vi "Z Aux Set Trace File.vi"(8 "error in (no error)":errorcluster caption="错误输入（无错误）", 10 "pFilePathName":string, 11 "bifTofile":i32) -> (0 "error out":errorcluster caption="错误输出", 3 "function return":i32)   [LabVIEW 2015, in "zauxdll.lvlib"]
doc: "int32 __stdcall ZAux_SetTraceFile(int bifTofile, const char *pFilePathName);"
uses:
  zauxdll.lvlib
  Radar - 2015 32bit_autoqueue_angle_0319/zauxdll-2014/zauxdll.dll
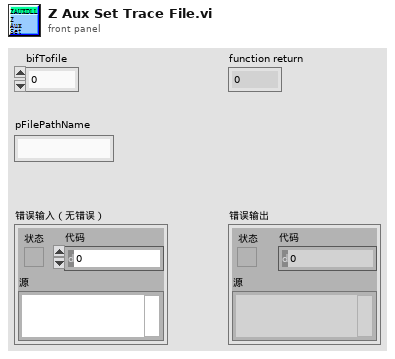
[diagram p1: front panel]
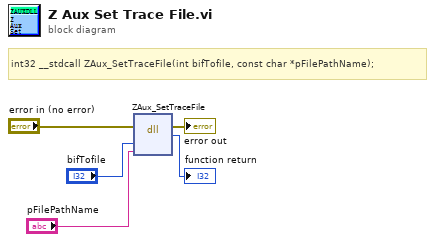
[diagram p0: block diagram]
diagram:
  # "int32 __stdcall ZAux_SetTraceFile(int bifTofile, const char *pFilePathName);"
  n1 = dll-call lib="D:/vicomm case/cub/0717/Radar - 2015 32bit_autoqueue_angle_0319/zauxdll-2014/zauxdll.*" fn="ZAux_SetTraceFile"(error in="error in (no error)", "bifTofile"="bifTofile", "pFilePathName"="pFilePathName") -> (error out=→"error out":errorcluster, →"function return":i32)  [unwired: 4 in, 1 out]
